vi "IDandCal.vi"(0 "ID列表In":string[](array[string]), 1 "数量统计in":string[](array[string]), 2 "ID输入":string, 3 "偏移量(0)":i32) -> (6 "ID列表":string[](array[string]), 7 "数量统计":string[](array[string]), 8 "ID输出":u32)   [LabVIEW 2015]
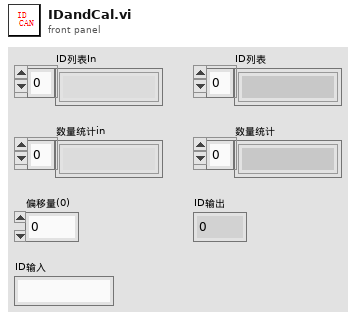
[diagram p1: front panel]
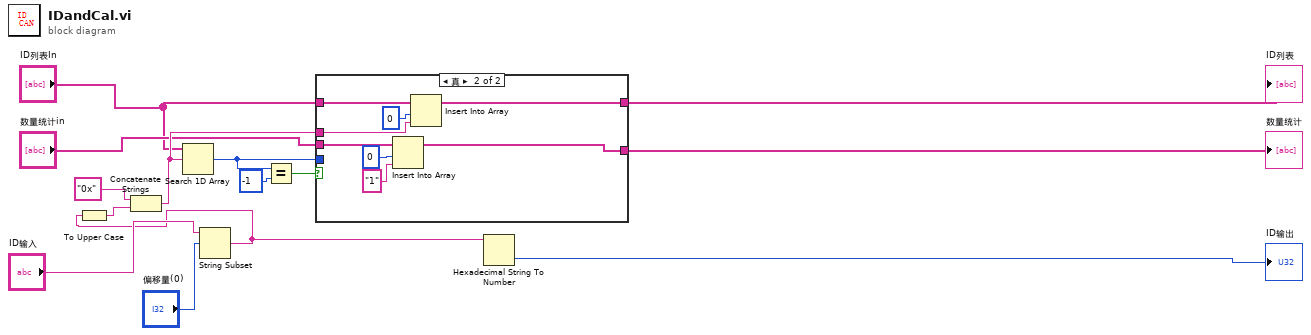
[diagram p0: block diagram]
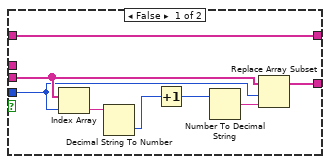
[diagram p2: hidden frame]
diagram:
  n1 = String Subset(string="ID输入", offset (0)="偏移量(0)") -> (substring=w13:string)  [unwired: 1 in]
  n2 = To Upper Case(1:w13) -> (0:w10:string)
  n3 = Concatenate Strings("0x" ("字符串"), w10) -> (w12:string)
  n4 = Search 1D Array(1D array="ID列表In", element=w12) -> (index of element=w8:i32)  [unwired: 1 in]
  n5 = Equal?(x=w8, y=-1) -> (x = y?=w4:bool)
  n6 = case shown="真" w4 {
    tunnel: "ID列表In" -> [w22 w30]
    tunnel: [w22 w29] -> w2
    tunnel: w12 -> [_ w28]
    tunnel: "数量统计in" -> [w21 w25]
    tunnel: [w20 w26] -> w7
    tunnel: w8 -> [w15 _]
    frame False {
      n7 = Index Array(array=w21, index=w15) -> (element=w19:string)
      n8 = Decimal String To Number(string=w19) -> (number=w18:i32)  [unwired: 2 in, 1 out]
      n9 = Increment(x=w18) -> (x+1=w16:i32)
      n10 = Number To Decimal String(number=w16) -> (decimal integer string=w17:string)  [unwired: 1 in]
      n11 = Replace Array Subset(array=w21, new element=w17, index=w15) -> (w20:string[])
    }
    frame True {
      n12 = Insert Into Array(array=w25, index=0 ("索引"), new element="1" ("新元素/子数组")) -> (w26:string[])
      n13 = Insert Into Array(array=w30, index=0 ("索引"), new element=w28) -> (w29:string[])
    }
  }
  "数量统计" <- w7
  "ID列表" <- w2
  n14 = Hexadecimal String To Number(string=w13) -> (number=→"ID输出":u32)  [unwired: 2 in, 1 out]
